vi "Main - Load Cell Calibration [Student].vi"() -> ()   [LabVIEW 2017]
uses:
  <vilib>/Utility/file.llb/Write To Spreadsheet File (DBL).vi
  <vilib>/ptbypt/NI_PtbyPt.lvlib
panel:
  out "10 Nuts":bool
  out "9 Nuts":bool
  out "8 Nuts":bool
  out "7 Nuts":bool
  out "6 Nuts":bool
  out "5 Nuts":bool
  out "4 Nuts":bool
  out "3 Nuts":bool
  out "2 Nuts":bool
  out "1 Nut":bool
  out "No Nuts":bool
  out "Data Table":cluster{"Force":dbl, "Voltage":dbl}[](array[cluster]) {"Force" format="%.3f"; "Voltage" format="%.4f"}
  out "Load Cell Voltage Characterisation":cluster{"X":dbl[], "Y":dbl[]}[](graph)
  out "Selected\nIndex":i32
  in  "Sample":bool
  in  "stop":bool
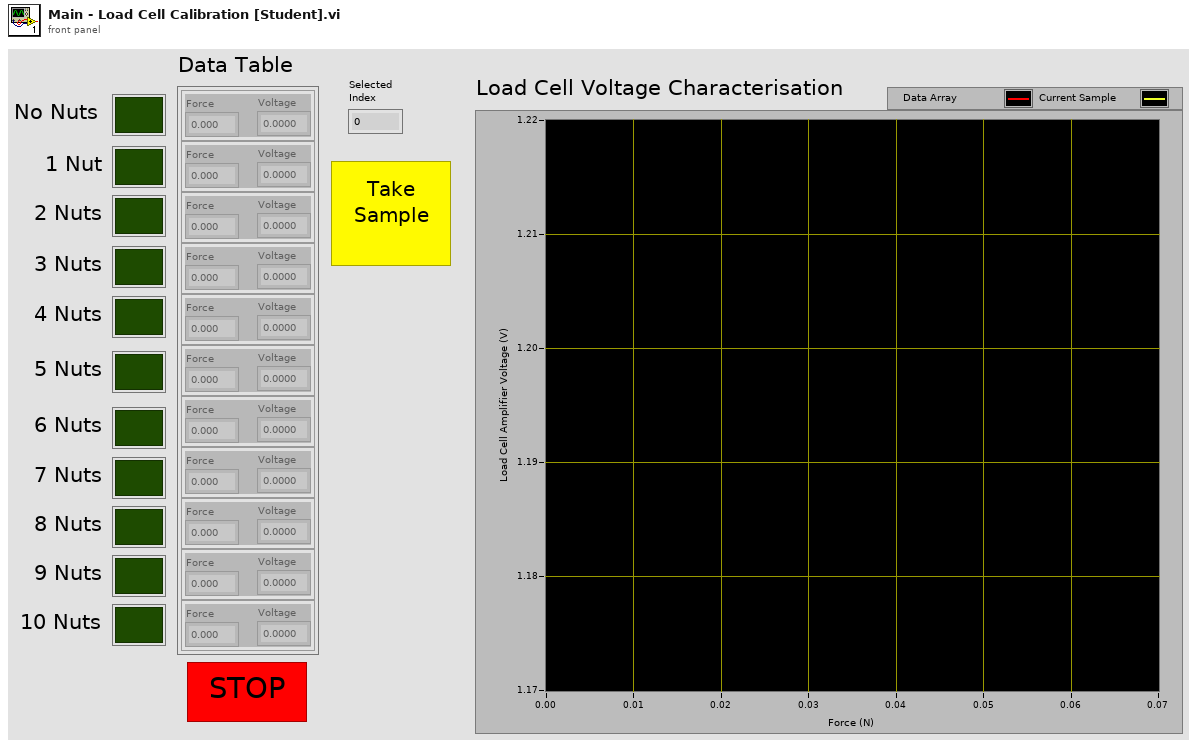
[diagram p1: front panel]
types:
  T1 = cluster{"AI Task":refnum<k21>, "Ctr0 Task":refnum<k21>, "Ao Task":refnum<k21>, "DO Task":refnum<k21>}
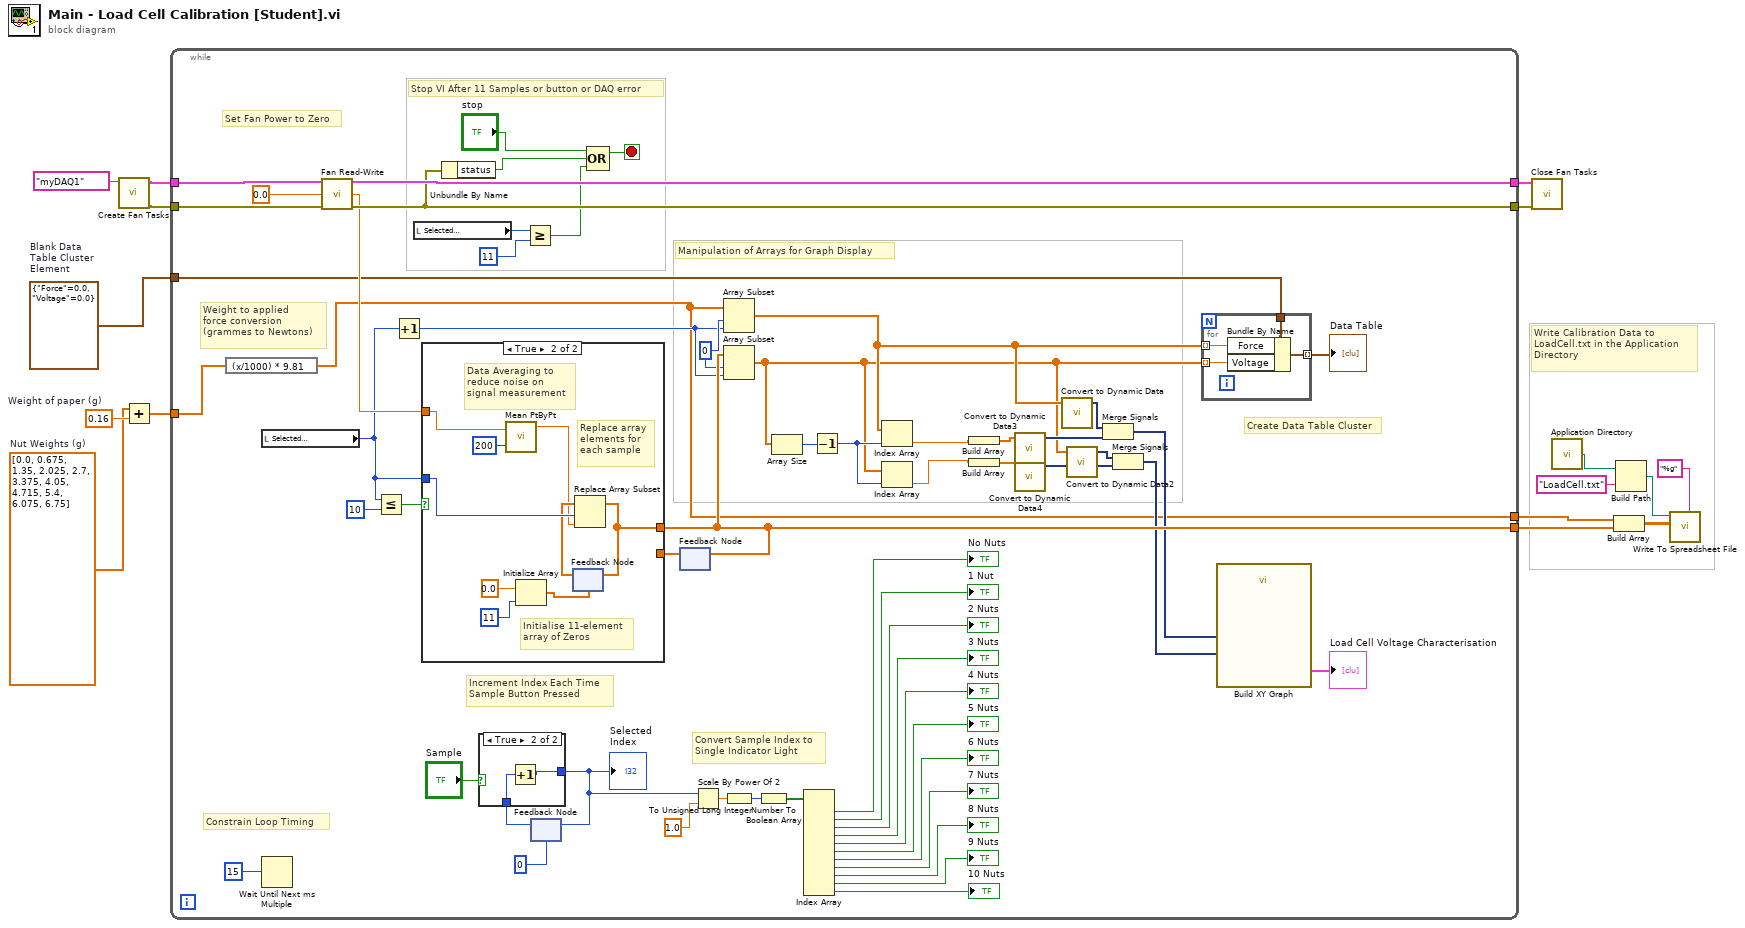
[diagram p0: block diagram]
diagram:
  w5 = 0.16  # Weight of paper (g)
  w3 = cluster{"Force":dbl, "Voltage":dbl} {"Force"=0.0, "Voltage"=0.0}  # Blank Data  Table Cluster  Element
  w4 = dbl[] [0.0, 0.675, 1.35, 2.025, 2.7, 3.375, 4.05, 4.715, 5.4, 6.075, 6.75]  # Nut Weights (g)
  # "Write Calibration Data to \nLoadCell.txt in the Application \nDirectory"
  n1 = call "Create Fan Tasks.vi"("DAQmx Device Name"=tag "myDAQ1") -> ("Error Out"=w15:errorcluster, "Hellicopter Tasks Output"=w16:T1)  [unwired: 5 in]
  n2 = Add(x=w4, y=w5) -> (x+y=w2:dbl[])
  n3 = while {
    tunnel: w15 -> [w72]
    tunnel: w16 -> [w73]
    tunnel: [w71] -> w13
    tunnel: [w70] -> w14
    tunnel: [w57] -> w6
    tunnel: w2 -> [w18]
    tunnel: w3 -> [w38]
    tunnel: [w17] -> w1
    stop <- w74 stop-if-true
    w56 = 0 ("index")
    # "Weight to applied\nforce conversion\n(grammes to Newtons)"
    # "Constrain Loop Timing"
    # "Create Data Table Cluster"
    # "Stop VI After 11 Samples or button or DAQ error"
    # "Manipulation of Arrays for Graph Display"
    # "Convert Sample Index to\nSingle Indicator Light"
    # "Increment Index Each Time\nSample Button Pressed"
    # "Set Fan Power to Zero"
    n4 = expression code="(x/1000) * 9.81"(w18) -> (w17:dbl[])
    n5 = local read "Selected\nIndex"() -> (w58:i32)
    n6 = Wait Until Next ms Multiple(millisecond multiple=u32 15) -> ()  [unwired: 1 out]
    n7 = call "Fan Read-Write.vi"("Hellicopter Tasks Input"=w73, "Fan Input"=0.0 ("Waveform"), "Error In"=w72) -> ("Hellicopter Tasks Output"=w71:T1, "L/C Output"=w66:dbl, "Error Out"=w70:errorcluster)  [unwired: 10 in]
    n8 = Less Or Equal?(x=w58, y=10) -> (x <= y?=w65:bool)
    n9 = Increment(x=w58) -> (x+1=w55:i32)
    n10 = local read "Selected\nIndex"() -> (w63:i32)
    n11 = Unbundle By Name(w70) -> ("status"=w21:bool)
    n12 = Greater Or Equal?(x=w63, y=11) -> (x >= y?=w62:bool)
    n13 = feedback #1(0 ("dimension size")) -> (w67:i32)
    n14 = case shown="True" "Sample" {
      tunnel: [w89 w90] -> w42
      tunnel: w67 -> [w89 w91]
      frame False {
      }
      frame True {
        n15 = Increment(x=w91) -> (x+1=w90:i32)
      }
    }
    "Selected\nIndex" <- w42
    n16 = feedback-in #1(w42) -> ()
    n17 = Compound Arithmetic op=OR("stop", w21, w62) -> (w74:bool)
    n18 = feedback #2() -> (w59:dbl[])  [unwired: 1 in]
    n19 = case shown="True" w65 {
      tunnel: w58 -> [_ w85]
      tunnel: w66 -> [_ w82]
      tunnel: [w79 w83] -> w57
      tunnel: w59 -> [w79 _]
      frame False {
      }
      frame True {
        # "Initialise 11-element \narray of Zeros"
        # "Replace array \nelements for \neach sample"
        # "Data Averaging to \nreduce noise on \nsignal measurement"
        n20 = call <vilib>:"Mean PtByPt.vi"("x"=w82, "sample length"=200) -> ("mean"=w81:dbl)  [unwired: 2 in, 1 out]
        n21 = Initialize Array(0.0 ("element"), 11 ("dimension size")) -> (w86:dbl[])
        n22 = feedback #3(w86) -> (w84:dbl[])
        n23 = Replace Array Subset(array=w84, new element=w81, index=w85) -> (w83:dbl[])
        n24 = feedback-in #3(w83) -> ()
      }
    }
    n25 = feedback-in #2(w57) -> ()
    n26 = Scale By Power Of 2(n=w42, x=1.0) -> (x*2^n=w41:dbl)
    n27 = Array Subset(array=w17, index=w56, length=w55) -> (w28:dbl[])
    n28 = Array Subset(array=w57, index=w56, length=w55) -> (w25:dbl[])
    n29 = To Unsigned Long Integer(number=w41) -> (unsigned 32bit integer=w39:u32)
    n30 = Number To Boolean Array(number=w39) -> (Boolean array=w40:bool[])
    n31 = Array Size(array=w25) -> (size(s)=w35:i32)
    n32 = Index Array(array=w40) -> (element #1=→"No Nuts":bool, element #2=→"1 Nut":bool, element #3=→"2 Nuts":bool, element #4=→"3 Nuts":bool, element #5=→"4 Nuts":bool, element #6=→"5 Nuts":bool, element #7=→"6 Nuts":bool, element #8=→"7 Nuts":bool, element #9=→"8 Nuts":bool, element #10=→"9 Nuts":bool, element #11=→"10 Nuts":bool)  [unwired: 11 in]
    n33 = Decrement(x=w35) -> (x-1=w34:i32)
    n34 = Index Array(array=w28, index=w34) -> (element=w33:dbl)
    n35 = Index Array(array=w25, index=w34) -> (element=w32:dbl)
    n36 = Build Array(w33) -> (w30:dbl[])
    n37 = Build Array(w32) -> (w31:dbl[])
    n38 = call "Convert to Dynamic Data3"("Array"=w30) -> ("Dynamic Data Type"=w29:dynamicdata)  [unwired: 3 in]
    n39 = call "Convert to Dynamic Data4"("Array"=w31) -> ("Dynamic Data Type"=w22:dynamicdata)  [unwired: 3 in]
    n40 = call "Convert to Dynamic Data"("Array"=w28) -> ("Dynamic Data Type"=w27:dynamicdata)  [unwired: 3 in]
    n41 = call "Convert to Dynamic Data2"("Array"=w25) -> ("Dynamic Data Type"=w23:dynamicdata)  [unwired: 3 in]
    n42 = Merge Signals(w27, w29) -> (w26:dynamicdata)
    n43 = Merge Signals(w23, w22) -> (w24:dynamicdata)
    n44 = for {
      tunnel: w25 -> [w76] mode=indexing
      tunnel: w28 -> [w77] mode=indexing
      tunnel: w38 -> [w78]
      tunnel: [w75] -> w37 mode=indexing
      n45 = Bundle By Name(cluster=w78, "Force"=w77, "Voltage"=w76) -> (w75:cluster{"Force":dbl, "Voltage":dbl})
    }
    "Data Table" <- w37
    n46 = call "Build XY Graph"("Y Input"=w24, "X Input"=w26) -> ("XY Graph"=→"Load Cell Voltage Characterisation":cluster{"X":dbl[], "Y":dbl[]}[])  [unwired: 8 in, 1 out]
  }
  n47 = call "Close Fan Tasks.vi"("Error In"=w14, "Hellicopter Tasks Input 2"=w13) -> ()  [unwired: 9 in, 1 out]
  n48 = call <vilib>:"Application Directory.vi"() -> ("Application Directory"=w11:path)
  n49 = Build Array(w1, w6) -> (w8:dbl[][])
  n50 = Build Path(base path=w11, name or relative path="LoadCell.txt") -> (appended path=w9:path)
  n51 = call-poly <vilib>:"Write To Spreadsheet File.vi"("format (%.3f)"="%g", "2D data"=w8, "file path (dialog if empty)"=w9) -> ()  [unwired: 5 in, 1 out]
